vi "arrayOfWaveforms.vi"() -> ()   [LabVIEW 2021]
panel:
  out "Waveform Graph":waveform(dbl)[](graph)
  in  "Array":waveform(dbl)[](array[waveform])
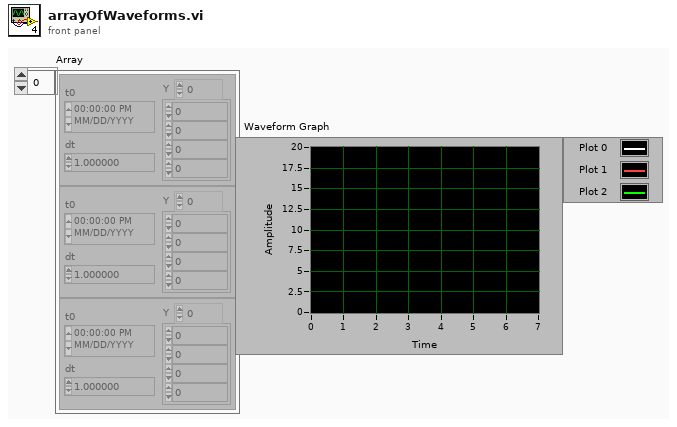
[diagram p1: front panel]
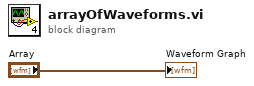
[diagram p0: block diagram]
diagram:
  "Waveform Graph" <- "Array"
